vi "General Error Handler Core CORE.vi"(0 "[error code] (0)":i32 format="%0.0f", 1 "[error source] (\" \")":string, 3 "String to Format (not a refnum)":refnum<vi>, 4 "type of dialog (OK msg:1)":T2=enum."OK message", 5 "error in (no error)":errorcluster, 6 "[user-defined codes]":i32[](array[numeric]), 7 "[exception action] (none:0)":i32(ring) items=["no exception", "cancel error on match", "set error on match"], 8 "ni.com link visible (F)":bool, 9 "prompts":T1={"Error %d occurred at %s"="Error %d occurred at %s", "Warning %d occurred at %s"="Warning %d occurred at %s", "Possible reasons: %s"="<b>Possible reason(s):</b>\\n%s", "Error not listed"="This error code is undefined. Undefined errors might occur for a number of reasons. For example, no one has provided a description for the code, or you might have wired a number that is not an error code to the error code input. \n\nAdditionally, undefined error codes might occur because the error relates to a third-party object, such as the operating system or ActiveX. For these third-party errors, you might be able to obtain a description of the error by searching the Web for the error code (%s) or for its hexadecimal representation (0x%s).", "GetCommError x%lx"="Windows GetCommError:  The hex value of this code is <B>x%04lx</B>.\n\nInterpret it bit-wise as follows:\n<B>x4000</B>: serial port VI error\n<B>x0001</B>: receiving queue overflowed or character was received after end-of-file character\n<B>x0002</B>: character was lost by overwrite\n<B>x0004</B>: parity error\n<B>x0008</B>: framing error\n<B>x0010</B>: break condition\n<B>x0020</B>: CTS timeout\n<B>x0040</B>: DSR timeout\n<B>x0080</B>: RLSD timeout\n<B>x0100</B>: transmission queue was full when new character arrived\n<B>x0200</B>: parallel device timeout\n<B>x0400</B>: parallel device I/O error\n<B>x0800</B>: parallel device not selected\n<B>x1000</B>: parallel device out of paper\n<B>x8000</B>: requested mode is  not supported or the idComDev parameter is invalid.", "Continue"="Continue", "Stop"="Stop", "an unidentified location"="an unidentified location", "No Error"="No Error", "Help"="Why not found?"}, 10 "[user-defined descriptions]":string[](array[string]), 11 "[exception code]":i32 format="%0.0f", 13 "[exception source]":string) -> (12 "stop event propagated":bool, 14 "error?":bool, 15 "code out":i32 format="%0.0f", 17 "source out":string, 18 "message":string=" INSTRUCTIONS:\r\rNormal Use:  When using subVIs that incorporate the error in/error out (or error I/O) structure, place this handler where you want to inform the user of an error, typically at the end of the I/O data path, as the last action of the program.  If the error in error? is ERROR, the handler creates a message describing the error and its source.  If the type of dialog = 1 (default), the message is displayed to the user, who can only acknowledge it.  If the type = 2, the user can acknowledge the message or abort execution; aborting a program with active I/O is not recommended.  If the type = 0, no message is displayed; this is used to process the error programmatically, and the error out cluster elements are wired to individual terminals for that reason.  \r\rOther Use:\n\r\nlocal testing.  To test the error code of a subVI or function that does not have the error I/O structure, you can wire its error code and a source string to the local error code and error source inputs.  If error in error? indicates no error and error code is not equal to 0, the local code and source are substituted for the error in values, and error? is set TRUE (ERROR).", 19 "error out":errorcluster)   [LabVIEW 2015]
doc: "Indicates whether an error occurred. If an error occurred, this VI returns a description of the error and optionally displays a dialog box."
uses:
  DialogTypeEnum.ctl
  whitespace.ctl
panel:
  # "reinitialize to default to display instructions"
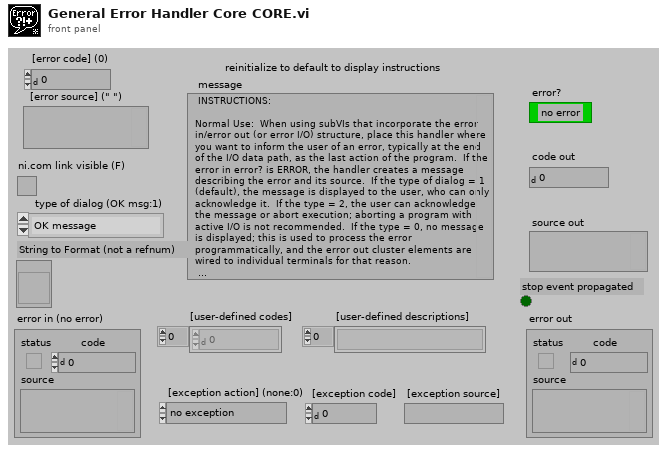
[diagram p1: front panel]
types:
  T1 = cluster{"Error %d occurred at %s":string, "Warning %d occurred at %s":string, "Possible reasons: %s":string, "Error not listed":string, "GetCommError x%lx":string, "Continue":string, "Stop":string, "an unidentified location":string, "No Error":string, "Help":string}
  T2 = typedef "DialogTypeEnum.ctl" = enum16{"no dialog", "OK message", "continue or stop message", "auto error handling dialog", "OK message + warnings", "continue/stop + warnings"}
  T3 = typedef "TagReturnType.ctl" = enum16{"No Tag", "<err>", "<append>"}
  T4 = typedef "whitespace.ctl" = u16
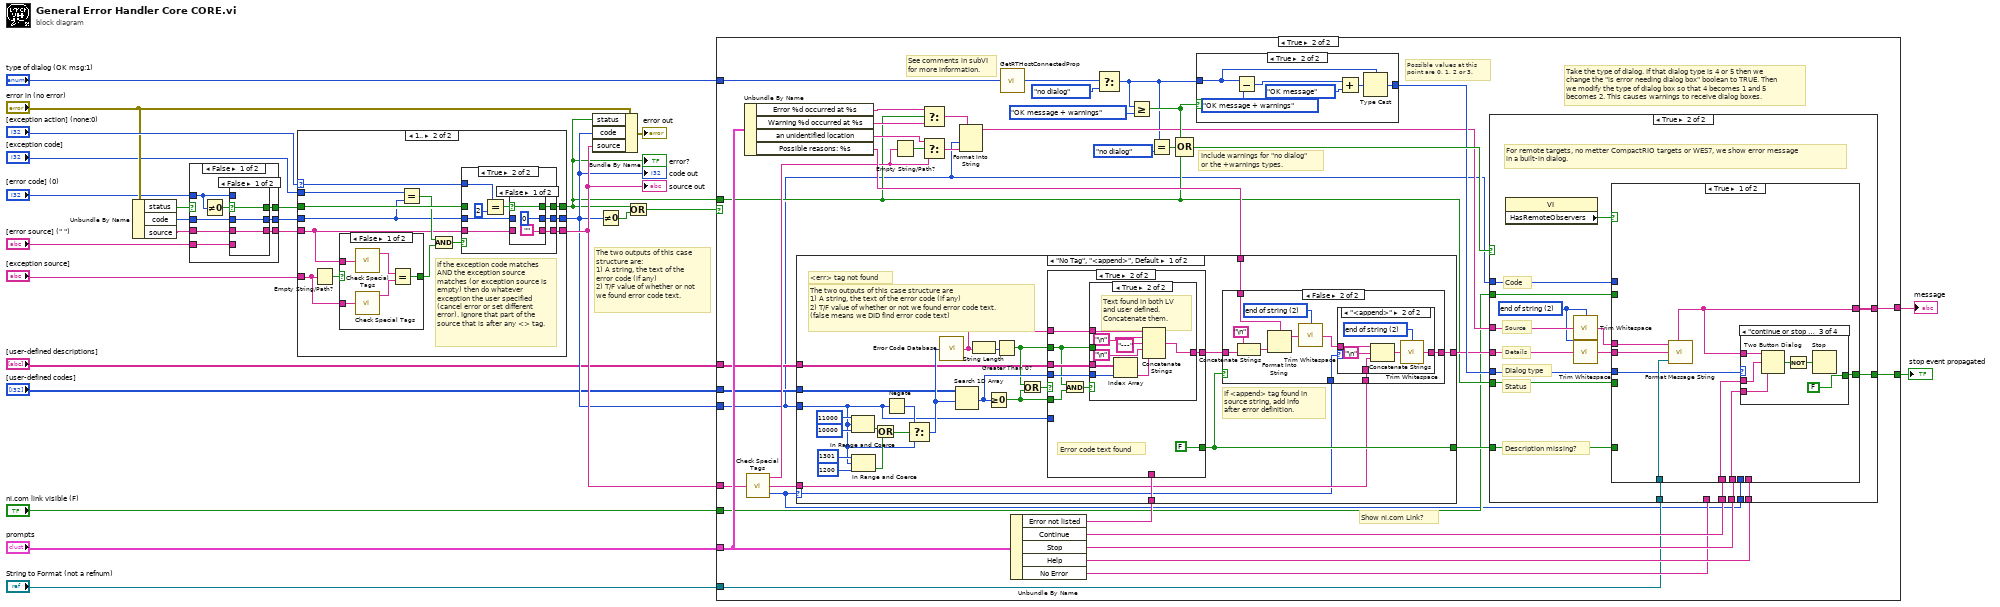
[diagram p0: block diagram]
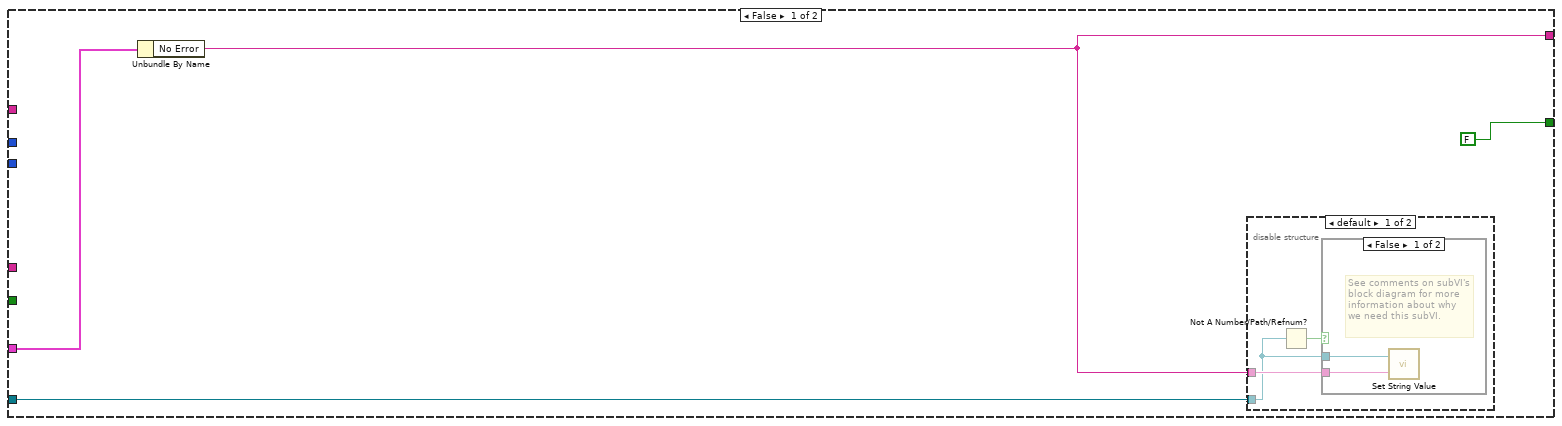
[diagram p8: hidden frame]
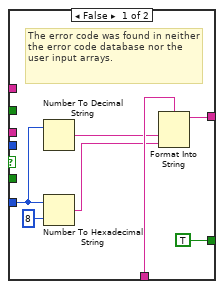
[diagram p14: hidden frame]
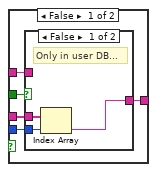
[diagram p15: hidden frame]
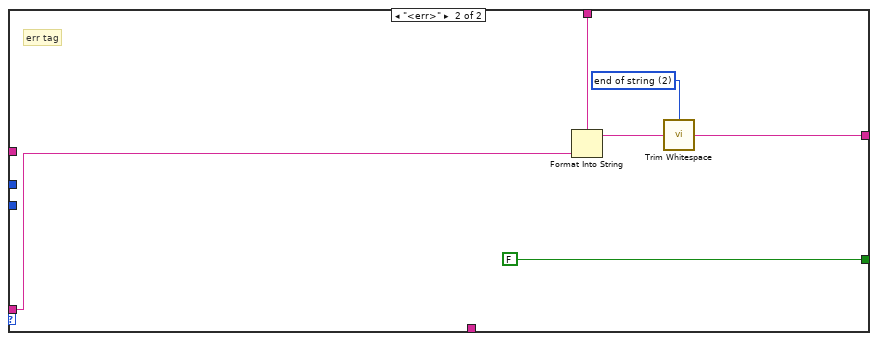
[diagram p17: hidden frame]
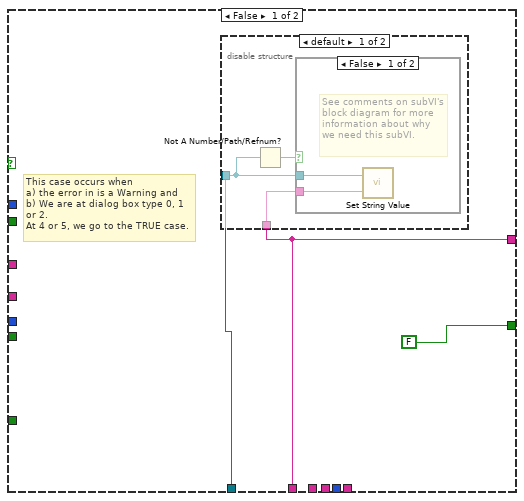
[diagram p18: hidden frame]
diagram:
  # "The two outputs of this case structure are:\n1) A string, the text of the error code (if any)\n2) T/F value of whether or not we found error code text."
  n1 = Unbundle By Name("error in (no error)") -> ("status"=w7:bool, "code"=w21:i32, "source"=w25:string)
  n2 = case shown="False" w7 {
    selector: w7 -> [_ w43]
    tunnel: [w32 w42] -> w23
    tunnel: [w33 w43] -> w22
    tunnel: w21 -> [w29 w42]
    tunnel: [w31 w41] -> w24
    tunnel: w25 -> [w30 w41]
    tunnel: "[error code] (0)" -> [w28 _]
    tunnel: "[error source] (\" \")" -> [w27 _]
    frame False {
      n3 = Not Equal To 0?(x=w28) -> (x != 0?=w34:bool)
      n4 = case shown="False" w34 {
        selector: w34 -> [w37 w40]
        tunnel: [w37 w40] -> w33
        tunnel: w28 -> [_ w39]
        tunnel: [w35 w39] -> w32
        tunnel: w27 -> [_ w38]
        tunnel: [w36 w38] -> w31
        tunnel: w30 -> [w36 _]
        tunnel: w29 -> [w35 _]
        frame False {
        }
        frame True {
        }
      }
    }
    frame True {
    }
  }
  n5 = case shown="1.." "[exception action] (none:0)" {
    selector: "[exception action] (none:0)" -> [_ w51]
    tunnel: [w46 w59] -> w3
    tunnel: w22 -> [w46 w57]
    tunnel: [w45 w58] -> w8
    tunnel: w23 -> [w45 w55]
    tunnel: [w44 w53] -> w18
    tunnel: w24 -> [w44 w49]
    tunnel: "[exception code]" -> [_ w52]
    tunnel: "[exception source]" -> [_ w48]
    frame ..0 {
    }
    frame 1.. {
      # "If the exception code matches AND the exception source matches (or exception source is empty) then do whatever exception the user specified (cancel error or set different error). Ignore that part of the source that is after any <> tag."
      n6 = Empty String/Path?(string/path=w48) -> (empty?=w50:bool)
      n7 = case shown="False" w50 {
        selector: w50 -> [_ w65]
        tunnel: w49 -> [w64 _]
        tunnel: w48 -> [w63 _]
        tunnel: [w62 w65] -> w47
        frame False {
          n8 = call "Check Special Tags.vi"("source"=w64) -> ("Before Tag (source)"=w61:string)  [unwired: 2 out]
          n9 = call "Check Special Tags.vi"("source"=w63) -> ("Before Tag (source)"=w60:string)  [unwired: 2 out]
          n10 = Equal?(x=w61, y=w60) -> (x = y?=w62:bool)
        }
        frame True {
          # "Empty string always matches."
        }
      }
      n11 = Equal?(x=w52, y=w55) -> (x = y?=w56:bool)
      n12 = And(x=w56, y=w47) -> (x .and. y?=w54:bool)
      n13 = case shown="True" w54 {
        tunnel: [w68 w69] -> w59
        tunnel: [w67 w73] -> w58
        tunnel: w57 -> [w68 _]
        tunnel: w55 -> [w67 w72]
        tunnel: w51 -> [_ w76]
        tunnel: [w66 w71] -> w53
        tunnel: w49 -> [w66 w70]
        frame False {
        }
        frame True {
          n14 = Equal?(x=w76, y=2) -> (x = y?=w74:bool)
          n15 = case shown="False" w74 {
            selector: w74 -> [w79 w82]
            tunnel: [0 w81] -> w73
            tunnel: w72 -> [_ w81]
            tunnel: ["" ("Empty String Constant") w80] -> w71
            tunnel: w70 -> [_ w80]
            tunnel: [w79 w82] -> w69
            frame False {
            }
            frame True {
            }
          }
        }
      }
    }
  }
  "source out" <- w18
  "error?" <- w3
  "code out" <- w8
  n16 = Bundle By Name(cluster="error in (no error)", "status"=w3, "code"=w8, "source"=w18) -> (→"error out":errorcluster)
  n17 = Not Equal To 0?(x=w8) -> (x != 0?=w2:bool)
  n18 = Or(x=w3, y=w2) -> (x .or. y?=w19:bool)
  n19 = case shown="True" w19 {
    tunnel: [w84 w112] -> w26
    tunnel: w3 -> [_ w95]
    tunnel: w18 -> [_ w102]
    tunnel: "prompts" -> [w86 w120]
    tunnel: [FALSE ("Stop 2") w115] -> w14
    tunnel: "String to Format (not a refnum)" -> [w83 w108]
    tunnel: w8 -> [_ w93]
    tunnel: "[user-defined descriptions]" -> [_ w99]
    tunnel: "[user-defined codes]" -> [_ w98]
    tunnel: "type of dialog (OK msg:1)" -> [_ w97]
    tunnel: "ni.com link visible (F)" -> [_ w94]
    frame False {
      n20 = Unbundle By Name(w86) -> ("No Error"=w84:string)
      n21 = disable-structure shown="default" {
        disable-tunnel: w84 -> [w89 _]
        disable-tunnel: w83 -> [w88 _]
        frame condition #0 {
          n22 = Not A Number/Path/Refnum?(number/path/refnum=w88) -> (NaN/Path/Refnum?=w87:bool)
          n23 = case shown="False" w87 {
            tunnel: w89 -> [w91 _]
            tunnel: w88 -> [w90 _]
            frame False {
              # "See comments on subVI's block diagram for more information about why we need this subVI."
              n24 = call "Set String Value.vi"("No Error"=w91, "String to Format (not a refnum)"=w90) -> ()
            }
            frame True {
            }
          }
        }
        frame condition #1 (active) {
          # "Do nothing in RT case."
        }
      }
    }
    frame True {
      # "Show ni.com Link?"
      # "See comments in subVI for more information."
      # "Include warnings for \"no dialog\" or the +warnings types."
      # "Possible values at this point are 0, 1, 2 or 3."
      # "Take the type of dialog. If that dialog type is 4 or 5 then we change the \"is error needing dialog box\" boolean to TRUE. Then we modify the type of dialog box so that 4 becomes 1 and 5 becomes 2. This causes warnings to receive dialog boxes."
      n25 = Unbundle By Name(w120) -> ("Error %d occurred at %s"=w100:string, "Warning %d occurred at %s"=w127:string, "an unidentified location"=w124:string, "Possible reasons: %s"=w114:string)
      n26 = call "Check Special Tags.vi"("source"=w102) -> ("Before Tag (source)"=w101:string, "After Tag (special data)"=w128:string, "Tag Found?"=w92:T3)
      n27 = Empty String/Path?(string/path=w101) -> (empty?=w129:bool)
      n28 = Select(t=w100, s=w95, f=w127) -> (s? t:f=w126:string)
      n29 = Select(t=w124, s=w129, f=w101) -> (s? t:f=w125:string)
      n30 = Format Into String(format string=w126, w93, w125) -> (resulting string=w110:string)  [unwired: 2 in, 1 out]
      n31 = call "GetRTHostConnectedProp.vi"() -> ("App.RTHostConnected"=w96:bool)
      n32 = Unbundle By Name(w120) -> ("Error not listed"=w123:string, "Continue"=w122:string, "Stop"=w121:string, "Help"=w118:string, "No Error"=w109:string)
      n33 = case shown="\"No Tag\", \"<append>\", Default" w92 {
        selector: w92 -> [w137 _]
        tunnel: [w142 w215] -> w111
        tunnel: w93 -> [w138 _]
        tunnel: w128 -> [w143 w214]
        tunnel: w123 -> [w161 _]
        tunnel: [w144 FALSE] -> w119
        tunnel: w114 -> [w146 w213]
        tunnel: w99 -> [w140 _]
        tunnel: w98 -> [w139 _]
        frame "No Tag", "<append>", Default {
          # "If <append> tag found in source string, add info after error definition."
          # "<err> tag not found"
          # "The two outputs of this case structure are\n1) A string, the text of the error code (if any)\n2) T/F value of whether or not we found error code text.\n(false means we DID find error code text)"
          n34 = In Range and Coerce(upper limit=11000, x=w138, lower limit=10000) -> (In Range?=w154:bool)  [unwired: 1 out]
          n35 = In Range and Coerce(upper limit=1301, x=w138, lower limit=1200) -> (In Range?=w155:bool)  [unwired: 1 out]
          n36 = Or(x=w154, y=w155) -> (x .or. y?=w153:bool)
          n37 = Negate(x=w138) -> (-x=w157:i32)
          n38 = Select(t=w157, s=w153, f=w138) -> (s? t:f=w141:i32)
          n39 = call "Error Code Database.vi"("Error Code"=w141) -> ("Error Text"=w147:string)
          n40 = Search 1D Array(1D array=w139, element=w141) -> (index of element=w160:i32)  [unwired: 1 in]
          n41 = String Length(string=w147) -> (length=w151:i32)
          n42 = Greater Or Equal To 0?(x=w160) -> (x >= 0?=w148:bool)
          n43 = Greater Than 0?(x=w151) -> (x > 0?=w149:bool)
          n44 = Or(x=w149, y=w148) -> (x .or. y?=w150:bool)
          n45 = case shown="True" w150 {
            tunnel: w160 -> [_ w190]
            tunnel: [w184 w188] -> w145
            tunnel: w161 -> [w183 _]
            tunnel: [TRUE FALSE] -> w144
            tunnel: w149 -> [_ w187]
            tunnel: w148 -> [_ w192]
            tunnel: w140 -> [_ w191]
            tunnel: w147 -> [_ w189]
            tunnel: w138 -> [w180 _]
            frame False {
              # "The error code was found in neither the error code database nor the user input arrays."
              n46 = Number To Decimal String(number=w180) -> (decimal integer string=w181:string)  [unwired: 1 in]
              n47 = Number To Hexadecimal String(1:i16 8 ("width (-)"), 2:w180) -> (0:w182:string)
              n48 = Format Into String(format string=w183, w181, w182) -> (resulting string=w184:string)  [unwired: 2 in, 1 out]
            }
            frame True {
              # "Error code text found"
              n49 = And(x=w187, y=w192) -> (x .and. y?=w193:bool)
              n50 = case shown="True" w193 {
                tunnel: w191 -> [w196 w211]
                tunnel: w190 -> [w195 w210]
                tunnel: w189 -> [w197 w204]
                tunnel: [w198 w208] -> w188
                tunnel: w187 -> [w199 _]
                frame False {
                  n51 = case shown="False" w199 {
                    tunnel: [w200 w203] -> w198
                    tunnel: w197 -> [_ w203]
                    tunnel: w196 -> [w202 _]
                    tunnel: w195 -> [w201 _]
                    frame False {
                      # "Only in user DB..."
                      n52 = Index Array(array=w202, index=w201) -> (element=w200:string)
                    }
                    frame True {
                      # "Only in LV DB..."
                    }
                  }
                }
                frame True {
                  # "Text found in both LV\nand user defined. \nConcatenate them."
                  n53 = Index Array(array=w211, index=w210) -> (element=w209:string)
                  n54 = Concatenate Strings(w204, "\n" ("End of Line Constant"), "---" ("string"), "\n" ("End of Line Constant"), w209) -> (w208:string)
                }
              }
            }
          }
          n55 = case shown="False" w144 {
            tunnel: w146 -> [_ w172]
            tunnel: [w162 w164] -> w142
            tunnel: w145 -> [w162 w169]
            tunnel: w137 -> [_ w166]
            tunnel: w143 -> [_ w165]
            frame True {
              # "no explanation given for error."
            }
            frame False {
              w163 = T4 2 items=["both", "start of string", "end of string"] ("location (both)")
              n56 = Concatenate Strings("\n" ("End of Line Constant"), w169) -> (w170:string)
              n57 = Format Into String(format string=w172, w170) -> (resulting string=w171:string)  [unwired: 2 in, 1 out]
              n58 = call "Trim Whitespace.vi"("string"=w171, "location (both)"=w163) -> ("trimmed string"=w167:string)
              n59 = case shown="\"<append>\"" w166 {
                tunnel: w167 -> [w173 w178]
                tunnel: [w173 w175] -> w164
                tunnel: w165 -> [_ w177]
                frame "No Tag", Default {
                }
                frame "<append>" {
                  w174 = T4 2 items=["both", "start of string", "end of string"] ("location (both)")
                  n60 = Concatenate Strings(w178, "\n" ("End of Line Constant"), w177) -> (w176:string)
                  n61 = call "Trim Whitespace.vi"("string"=w176, "location (both)"=w174) -> ("trimmed string"=w175:string)
                }
              }
            }
          }
        }
        frame "<err>" {
          w212 = T4 2 items=["both", "start of string", "end of string"] ("location (both)")
          # "err tag"
          n62 = Format Into String(format string=w213, w214) -> (resulting string=w216:string)  [unwired: 2 in, 1 out]
          n63 = call "Trim Whitespace.vi"("string"=w216, "location (both)"=w212) -> ("trimmed string"=w215:string)
        }
      }
      n64 = Select(t=w97, s=w96, f=DialogTypeEnum."no dialog" ("type of dialog (OK msg:1)")) -> (s? t:f=w103:T2)
      n65 = Greater Or Equal?(x=w103, y=DialogTypeEnum."OK message + warnings" ("type of dialog (OK msg:1)")) -> (x >= y?=w116:bool)
      n66 = Equal?(x=w103, y=DialogTypeEnum."no dialog" ("type of dialog (OK msg:1)")) -> (x = y?=w107:bool)
      n67 = Compound Arithmetic op=OR(w116, w107, w95) -> (w117:bool)
      n68 = case shown="True" w116 {
        tunnel: w103 -> [w130 w131]
        tunnel: [w130 w133] -> w113
        frame False {
        }
        frame True {
          n69 = Subtract(x=w131, y=DialogTypeEnum."OK message + warnings" ("type of dialog (OK msg:1)")) -> (x-y=w136:u16)
          n70 = Add(x=w136, y=DialogTypeEnum."OK message" ("type of dialog (OK msg:1)")) -> (x+y=w132:u16)
          n71 = Type Cast(type=w131, x=w132) -> (*(type *) &x=w133:T2)
        }
      }
      n72 = case shown="True" w117 {
        tunnel: w113 -> [_ w243]
        tunnel: w122 -> [_ w242]
        tunnel: w121 -> [_ w241]
        tunnel: w119 -> [_ w230]
        tunnel: w118 -> [_ w240]
        tunnel: w110 -> [_ w233]
        tunnel: w111 -> [_ w234]
        tunnel: w95 -> [_ w239]
        tunnel: [FALSE ("Stop 2") w238] -> w115
        tunnel: [w218 w237] -> w112
        tunnel: w109 -> [w218 _]
        tunnel: w108 -> [w219 w236]
        tunnel: w94 -> [_ w228]
        tunnel: w93 -> [_ w229]
        tunnel: w92 -> [_ w227]
        frame False {
          # "This case occurs when\na) the error in is a Warning and\nb) We are at dialog box type 0, 1 or 2.\nAt 4 or 5, we go to the TRUE case."
          n73 = disable-structure shown="default" {
            disable-tunnel: w219 -> [w223 _]
            disable-tunnel: w218 -> [w221 _]
            frame condition #0 {
              n74 = Not A Number/Path/Refnum?(number/path/refnum=w223) -> (NaN/Path/Refnum?=w222:bool)
              n75 = case shown="False" w222 {
                tunnel: w221 -> [w225 _]
                tunnel: w223 -> [w224 _]
                frame False {
                  # "See comments on subVI's block diagram for more information about why we need this subVI."
                  n76 = call "Set String Value.vi"("No Error"=w225, "String to Format (not a refnum)"=w224) -> ()
                }
                frame True {
                }
              }
            }
            frame condition #1 (active) {
              # "Do nothing in RT case."
            }
          }
        }
        frame True {
          w231 = T4 2 items=["both", "start of string", "end of string"] ("location (both)")
          # "For remote targets, no metter CompactRIO targets or WES7, we show error message \nin a built-in dialog."
          # "Code"
          # "Description missing?"
          # "Dialog type"
          # "Status"
          # "Details"
          # "Source"
          n77 = property class="VI"() -> ("HasRemoteObservers"=w226:bool)  [unwired: 2 in, 2 out]
          n78 = call "Trim Whitespace.vi"("string"=w233, "location (both)"=w231) -> ("trimmed string"=w232:string)
          n79 = call "Trim Whitespace.vi"("string"=w234, "location (both)"=w231) -> ("trimmed string"=w235:string)
          n80 = case shown="True" w226 {
            tunnel: w243 -> [w244 w280]
            tunnel: w242 -> [w248 w279]
            tunnel: w241 -> [w247 w278]
            tunnel: w240 -> [_ w277]
            tunnel: w239 -> [_ w276]
            tunnel: [w246 w275] -> w238
            tunnel: [w245 w274] -> w237
            tunnel: w236 -> [w249 w273]
            tunnel: w235 -> [w250 w272]
            tunnel: w232 -> [w251 w271]
            tunnel: w230 -> [_ w270]
            tunnel: w229 -> [_ w269]
            tunnel: w228 -> [_ w268]
            tunnel: w227 -> [_ w267]
            frame True {
              n81 = call "Format Message String.vi"("Source"=w251, "Details"=w250, "String to Format (not a refnum)"=w249) -> ("message"=w245:string)  [unwired: 1 in, 4 out]
              n82 = case shown="\"continue or stop message\", \"continue/stop + warnings\"" w244 {
                tunnel: [FALSE ("stop event propagated") FALSE ("stop event propagated") FALSE ("stop event propagated") w262] -> w246
                tunnel: w245 -> [_ w254 w261 w266]
                tunnel: w248 -> [_ w253 w260 w265]
                tunnel: w247 -> [_ _ w259 w264]
                frame "no dialog" {
                }
                frame "OK message", "OK message + warnings", Default {
                  n83 = One Button Dialog(message=w254, button name ("OK")=w253) -> ()  [unwired: 1 out]
                }
                frame "continue or stop message", "continue/stop + warnings" {
                  n84 = Two Button Dialog(message=w261, 1:w259, 2:w260) -> (T button?=w257:bool)
                  n85 = Not(x=w257) -> (.not. x?=w256:bool)
                  n86 = Stop(stop? (T)=w256) -> ()
                }
                frame "auto error handling dialog" {
                  n87 = Two Button Dialog(message=w266, 1:w264, 2:w265) -> (T button?=w263:bool)
                  n88 = Not(x=w263) -> (.not. x?=w262:bool)
                }
              }
            }
            frame False {
              n89 = disable-structure "Conditional Disable Structure" shown="TARGET_TYPE==RT" {
                disable-tunnel: w280 -> [w294 _]
                disable-tunnel: w279 -> [w293 _]
                disable-tunnel: w278 -> [w292 _]
                disable-tunnel: w277 -> [w291 _]
                disable-tunnel: w276 -> [w290 _]
                disable-tunnel: [w289 FALSE ("stop event propagated")] -> w275
                disable-tunnel: [w288 "" ("message")] -> w274
                disable-tunnel: w273 -> [w287 _]
                disable-tunnel: w272 -> [w286 _]
                disable-tunnel: w271 -> [w285 _]
                disable-tunnel: w270 -> [w284 _]
                disable-tunnel: w268 -> [w282 _]
                disable-tunnel: w269 -> [w283 _]
                disable-tunnel: w267 -> [w281 _]
                frame condition #0 {
                  n90 = case shown="True" w284 {
                    tunnel: w286 -> [w309 w328]
                    tunnel: w291 -> [_ w334]
                    tunnel: w293 -> [w305 w332]
                    tunnel: w292 -> [w304 w331]
                    tunnel: w294 -> [w307 w333]
                    tunnel: [w306 w330] -> w289
                    tunnel: w285 -> [w310 w329]
                    tunnel: w290 -> [w303 _]
                    tunnel: [w298 w326] -> w288
                    tunnel: w287 -> [w308 w324]
                    tunnel: w282 -> [w296 _]
                    tunnel: w283 -> [w297 _]
                    tunnel: w281 -> [w295 _]
                    frame False {
                      n91 = call "Format Message String.vi"("Source"=w310, "Details"=w309, "String to Format (not a refnum)"=w308) -> ("message"=w298:string, "Bold Start"=w302:i32[], "Bold Length"=w301:i32[], "Source Out"=w300:string, "Details Out"=w299:string)  [unwired: 1 in]
                      n92 = case shown="\"OK message\", Default" w307 {
                        selector: w307 -> [_ w320]
                        tunnel: [FALSE ("stop event propagated") w323] -> w306
                        tunnel: w305 -> [_ w321]
                        tunnel: w304 -> [_ w322]
                        tunnel: w303 -> [_ w319]
                        tunnel: w302 -> [_ w315]
                        tunnel: w301 -> [_ w318]
                        tunnel: w300 -> [_ w317]
                        tunnel: w299 -> [_ w316]
                        tunnel: w296 -> [_ w314]
                        tunnel: w297 -> [_ w313]
                        tunnel: w295 -> [_ w312]
                        frame "no dialog" {
                        }
                        frame "OK message", Default {
                          n93 = call "Details Display Dialog.vi"("Source"=w317, "Start"=w315, "Length"=w318, "code"=w313, "Show Link"=w314, "Details"=w316, "dialog type"=w320, "Error or Warning"=w319, "contname"=w321, "stopname"=w322, "okname"=w321, "Tag Found?"=w312) -> ("stop event propagated"=w323:bool)  [unwired: 3 in]
                        }
                      }
                    }
                    frame True {
                      w327 = "\n" ("End of Line Constant")
                      n94 = Concatenate Strings(w329, w327, w327, w328) -> (w326:string)
                      n95 = Not A Number/Path/Refnum?(number/path/refnum=w324) -> (NaN/Path/Refnum?=w325:bool)
                      n96 = call "Not Found Dialog.vi"("Help"=w334, "Message"=w326, "Stop"=w331, "Continue"=w332, "type of dialog (OK msg:1)"=w333) -> ("stop event propagated"=w330:bool)  [unwired: 1 in]
                      n97 = case shown="True" w325 {
                        tunnel: w324 -> [w336 _]
                        tunnel: w326 -> [w335 _]
                        frame False {
                          n98 = call "Set String Value.vi"("No Error"=w335, "String to Format (not a refnum)"=w336) -> ()
                        }
                        frame True {
                        }
                      }
                    }
                  }
                }
                frame condition #1 (active) {
                }
              }
            }
          }
        }
      }
    }
  }
  "message" <- w26
  "stop event propagated" <- w14
